vi "ReadAll.vi"(8 "error in (no error)":errorcluster, 11 "VXMCfg in":refnum<class "VXMCfg.lvclass">) -> (0 "error out":errorcluster, 1 "VXM Properties.sub-syst.3":T1, 2 "VXM Properties.sub-syst.2":T1, 3 "VXMCfg out":refnum<class "VXMCfg.lvclass">, 5 "VXM Properties.sub-syst.1":T1)   [LabVIEW 2018, in "VXMCfg.lvclass"]
uses:
  VXMCfg.lvclass
  sub-syst.n.ctl
  VXMCfg.lvclass/VXMCfg.ctl
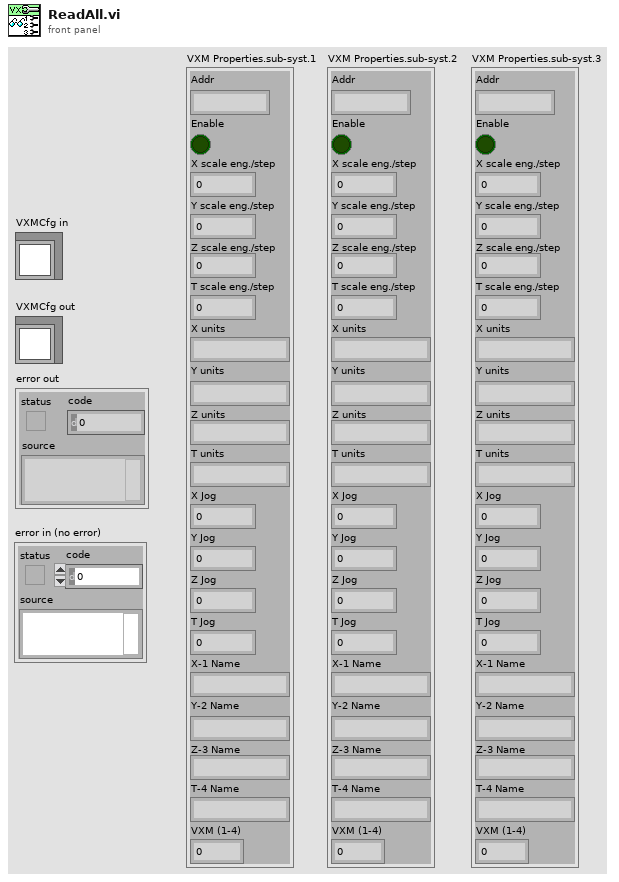
[diagram p1: front panel]
types:
  T1 = typedef "sub-syst.n.ctl" = cluster{"Addr":string, "Enable":bool, "X scale eng./step":dbl, "Y scale eng./step":dbl, "Z scale eng./step":dbl, "T scale eng./step":dbl, "X units":string, "Y units":string, "Z units":string, "T units":string, "X Jog":dbl, "Y Jog":dbl, "Z Jog":dbl, "T Jog":dbl, "X-1 Name":string, "Y-2 Name":string, "Z-3 Name":string, "T-4 Name":string, "VXM (1-4)":i32}
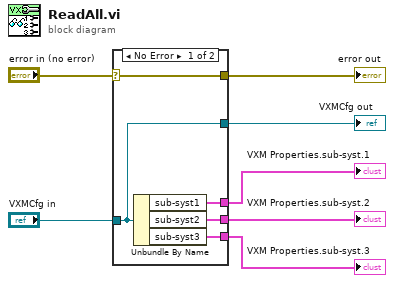
[diagram p0: block diagram]
diagram:
  n1 = case shown="No Error" "error in (no error)" {
    selector: "error in (no error)" -> [w12 w14]
    tunnel: [w12 w14] -> w6
    tunnel: [w11 w13] -> w4
    tunnel: "VXMCfg in" -> [w11 w13]
    tunnel: [w10 _] -> w3
    tunnel: [w9 _] -> w2
    tunnel: [w8 _] -> w1
    frame No Error {
      n2 = Unbundle By Name(w11) -> ("sub-syst1"=w8:T1, "sub-syst2"=w9:T1, "sub-syst3"=w10:T1)
    }
    frame Error {
    }
  }
  "error out" <- w6
  "VXMCfg out" <- w4
  "VXM Properties.sub-syst.1" <- w1
  "VXM Properties.sub-syst.2" <- w2
  "VXM Properties.sub-syst.3" <- w3
